vi "Interpolation.vi"(9 "Real Data":dbl[](array[numeric]), 10 "Lower Limit":dbl[](array[numeric]), 11 "Upper Limit":dbl[](array[numeric])) -> (3 "instances of true":dbl)   [LabVIEW 2014]
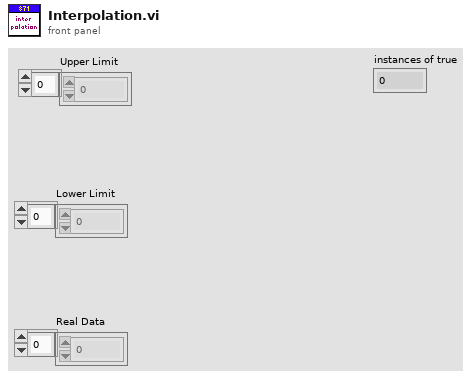
[diagram p1: front panel]
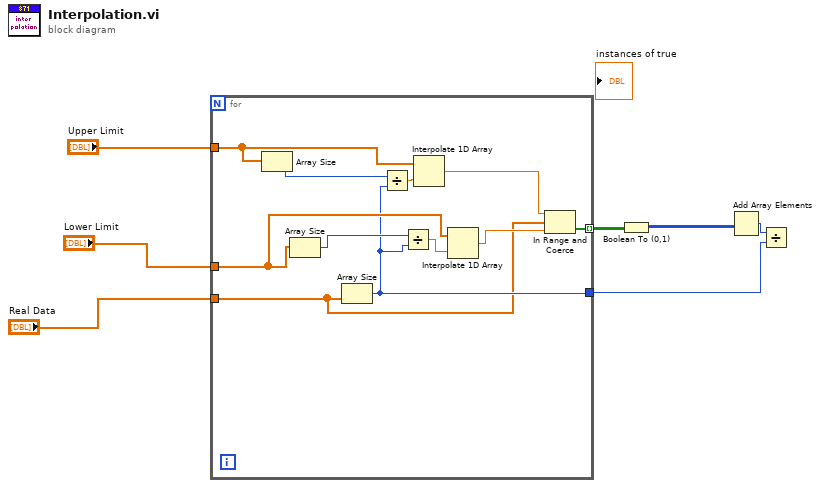
[diagram p0: block diagram]
diagram:
  n1 = for {
    tunnel: "Real Data" -> [w9]
    tunnel: "Upper Limit" -> [w16]
    tunnel: "Lower Limit" -> [w13]
    tunnel: [w12] -> w2
    tunnel: [w8] -> w1 mode=indexing
    n2 = Array Size(array=w16) -> (size(s)=w18:i32)
    n3 = Array Size(array=w13) -> (size(s)=w15:i32)
    n4 = Array Size(array=w9) -> (size(s)=w12:i32)
    n5 = Divide(x=w18, y=w12) -> (x/y=w17:dbl)
    n6 = Divide(x=w15, y=w12) -> (x/y=w14:dbl)
    n7 = Interpolate 1D Array(1:w17, 2:w16) -> (0:w11:dbl)
    n8 = Interpolate 1D Array(1:w14, 2:w13) -> (0:w10:dbl)
    n9 = In Range and Coerce(upper limit=w11, x=w9, lower limit=w10) -> (In Range?=w8:bool[])  [unwired: 1 out]
  }
  n10 = Boolean To (0,1)(Boolean=w1) -> (0, 1=w4:i16[][])
  n11 = Add Array Elements(numeric array=w4) -> (sum=w3:i16)
  n12 = Divide(x=w3, y=w2) -> ()  [unwired: 1 out]
